vi "create node.vi"(7 "unique name (false)":bool, 8 "error in":errorcluster, 10 "buffer size (-1, unlimited)":i32=-1, 11 "node name":string) -> (0 "error out":errorcluster, 3 "node ref out":T1)   [LabVIEW 2020, in "Publisher Subscriber.lvlib"]
doc: "Creates a new node in the project. Set the \"unique name\" value to TRUE when used to template modules. That will create unique name for every template."
uses:
  Publisher Subscriber.lvlib
  Controls/node refnum.ctl
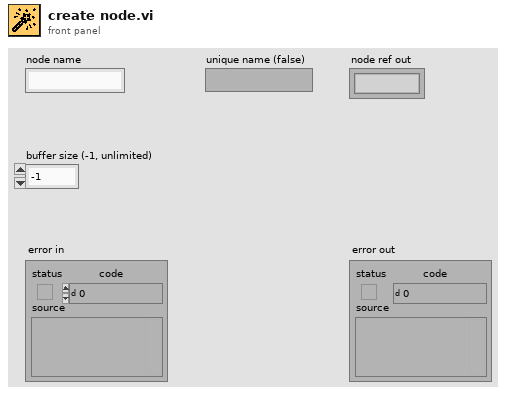
[diagram p1: front panel]
types:
  T1 = typedef "Publisher Subscriber.lvlib/node refnum.ctl" = refnum<k1>
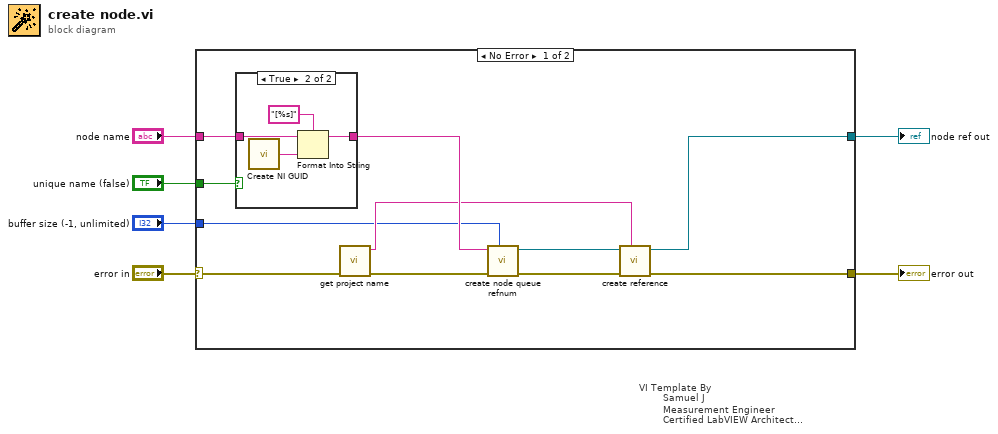
[diagram p0: block diagram]
diagram:
  n1 = case "VI Template By\n        Samuel J\n        Measurement Engineer\n        Certified LabVIEW Architect\n        Vestas Technology R&D Chennai" shown="No Error" "error in" {
    selector: "error in" -> [w17 w23]
    tunnel: [w14 w23] -> w5
    tunnel: "node name" -> [w10 _]
    tunnel: [w12 _] -> w3
    tunnel: "unique name (false)" -> [w9 _]
    tunnel: "buffer size (-1, unlimited)" -> [w7 _]
    frame No Error {
      n2 = case shown="True" w9 {
        tunnel: [w18 w22] -> w11
        tunnel: w10 -> [w18 w21]
        frame False {
        }
        frame True {
          n3 = call <vilib>:"Create NI GUID.vi"() -> ("NI GUID"=w20:string)
          n4 = Format Into String(format string="[%s]", initial string=w21, w20) -> (resulting string=w22:string)  [unwired: 1 in, 1 out]
        }
      }
      n5 = call "get project name.vi"("error in (no error)"=w17) -> ("error out"=w16:errorcluster, "Project name"=w8:string)  [unwired: 9 in]
      n6 = call "create node queue refnum.vi"("buffer size (-1, unlimited)"=w7, "error in"=w16, "Subscriber name"=w11) -> ("error out"=w13:errorcluster, "queue out"=w15:refnum<queue>)  [unwired: 7 in]
      n7 = call "create reference.vi"("project name"=w8, "error in"=w13, "queue ref"=w15) -> ("error out"=w14:errorcluster, "node ref"=w12:T1)  [unwired: 7 in]
    }
    frame Error {
    }
  }
  "error out" <- w5
  "node ref out" <- w3
